vi "GFITS_buildNextImageName.vi"(7 "incnumber":bool=TRUE, 8 "set dbs":bool=TRUE, 9 "Database RefNum":T1) -> (1 "image path":string)   [LabVIEW 2016]
uses:
  DBSHAND/private/vis/DatabaseHand_RefNum.ctl
  DBSHAND/private/vis/DatabaseHand_Element_Get(bool).vi
  DBSHAND/private/vis/DatabaseHand_Element_Get(string).vi
  DBSHAND/private/vis/DatabaseHand_Element_Set(I32).vi
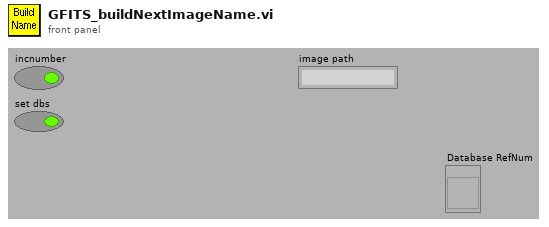
[diagram p1: front panel]
types:
  T1 = typedef "DatabaseHand_RefNum.ctl" = refnum<vi>
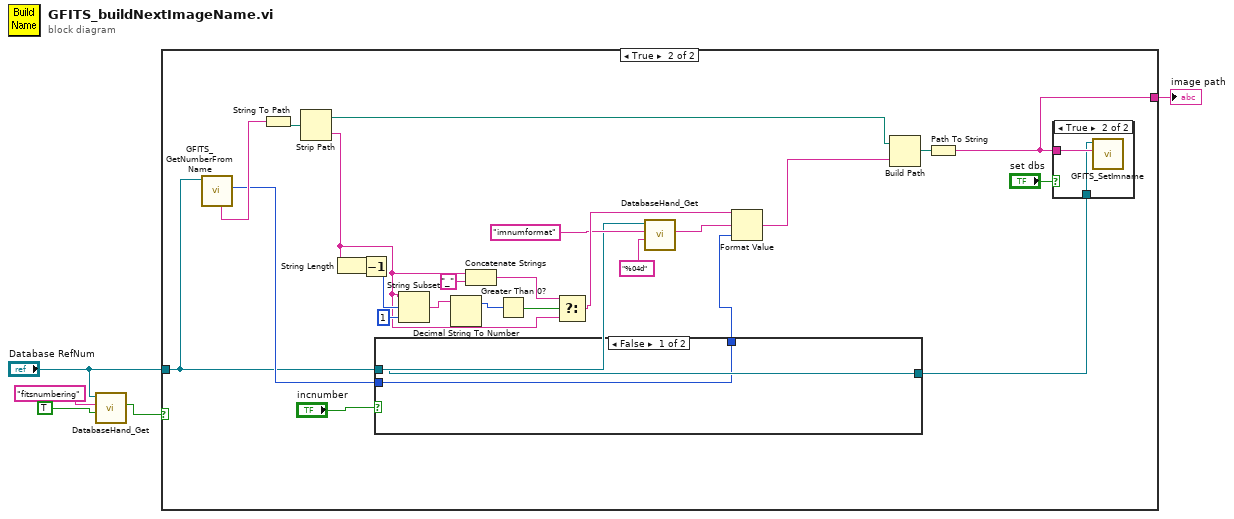
[diagram p0: block diagram]
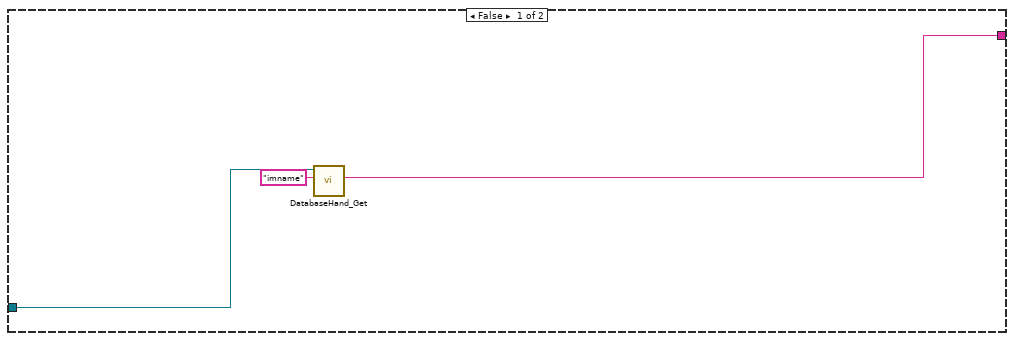
[diagram p2: hidden frame]
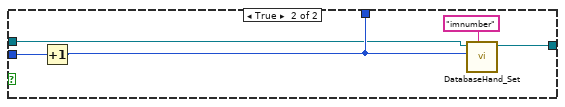
[diagram p4: hidden frame]
diagram:
  n1 = call-poly "DatabaseHand_Get.vi"("default value"=TRUE, "name"="fitsnumbering", "Database RefNum in"="Database RefNum") -> ("value"=w2:bool)  [unwired: 2 in, 6 out]
  n2 = case shown="True" w2 {
    tunnel: "Database RefNum" -> [w8 w12]
    tunnel: [w6 w9] -> w1
    frame False {
      n3 = call-poly "DatabaseHand_Get.vi"("name"="imname", "Database RefNum in"=w8) -> ("value"=w6:string)  [unwired: 3 in, 6 out]
    }
    frame True {
      n4 = call "GFITS_GetNumberFromName.vi"("Database RefNum in"=w12) -> ("number"=w16:i32, "rootname"=w17:string)  [unwired: 1 in, 8 out]
      n5 = String To Path(string=w17) -> (path=w32:path)
      n6 = Strip Path(path=w32) -> (stripped path=w13:path, name=w18:string)
      n7 = String Length(string=w18) -> (length=w31:i32)
      n8 = Decrement(x=w31) -> (x-1=w23:i32)
      n9 = case shown="False" "incnumber" {
        tunnel: [w37 w41] -> w19
        tunnel: w16 -> [w36 w40]
        tunnel: [w36 w39] -> w15
        tunnel: w12 -> [w37 w38]
        frame False {
        }
        frame True {
          n10 = Increment(x=w40) -> (x+1=w39:i32)
          n11 = call-poly "DatabaseHand_Set.vi"("name"="imnumber", "value"=w39, "Database RefNum in"=w38) -> ("Database RefNum out"=w41:T1)  [unwired: 5 in, 3 out]
        }
      }
      n12 = String Subset(string=w18, offset (0)=w23, length (rest)=1 ("length (rest)")) -> (substring=w29:string)
      n13 = Decimal String To Number(string=w29) -> (offset past number=w28:i32)  [unwired: 3 out]
      n14 = Concatenate Strings(w18, "_" ("string")) -> (w25:string)
      n15 = Greater Than 0?(x=w28) -> (x > 0?=w27:bool)
      n16 = Select(t=w25, s=w27, f=w18) -> (s? t:f=w24:string)
      n17 = call-poly "DatabaseHand_Get.vi"("default value"="%04d" ("format string"), "name"="imnumformat", "Database RefNum in"=w12) -> ("value"=w20:string)  [unwired: 2 in, 6 out]
      n18 = Format Value(string ("")=w24, format string=w20, value (0)=w15) -> (output string=w33:string)
      n19 = Build Path(base path=w13, name or relative path=w33) -> (appended path=w14:path)
      n20 = Path To String(path=w14) -> (string=w9:string)
      n21 = case shown="True" "set dbs" {
        tunnel: w9 -> [_ w35]
        tunnel: w19 -> [_ w34]
        frame False {
        }
        frame True {
          n22 = call "GFITS_SetImname.vi"("name"=w35, "Database RefNum"=w34) -> ()  [unwired: 1 in, 9 out]
        }
      }
    }
  }
  "image path" <- w1
